vi "Write Name.vi"(8 "error in (no error)":errorcluster, 10 "Name":string, 11 "Stop Response Msg in":refnum<class "Stop Response Msg.lvclass">) -> (0 "error out":errorcluster, 3 "Stop Response Msg out":refnum<class "Stop Response Msg.lvclass">)   [LabVIEW 2016, in "Stop Response Msg.lvclass"]
uses:
  Stop Response Msg.lvclass
  Stop Response Msg.lvclass/Stop Response Msg.ctl
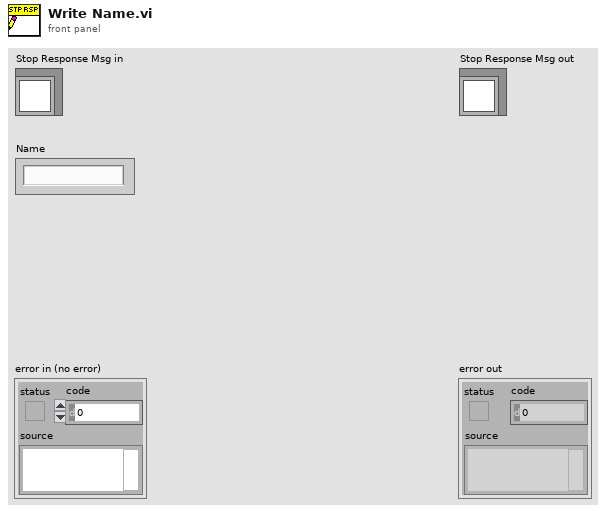
[diagram p1: front panel]
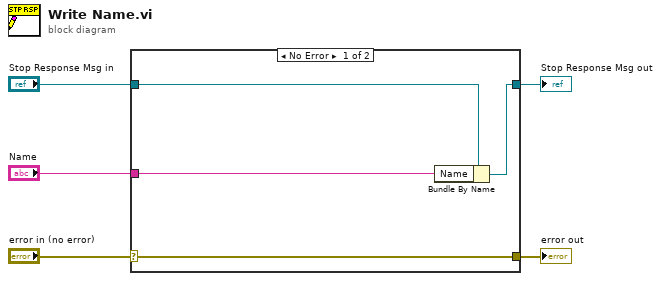
[diagram p0: block diagram]
diagram:
  n1 = case shown="No Error" "error in (no error)" {
    selector: "error in (no error)" -> [w9 w10]
    tunnel: [w9 w10] -> w4
    tunnel: [w7 w11] -> w2
    tunnel: "Stop Response Msg in" -> [w8 w11]
    tunnel: "Name" -> [w6 _]
    frame No Error {
      n2 = Bundle By Name(cluster=w8, "Name"=w6) -> (w7:refnum<class "Stop Response Msg.lvclass">)
    }
    frame Error {
    }
  }
  "error out" <- w4
  "Stop Response Msg out" <- w2
